vi "Read Index.vi"(3 "Index_Pointer)":refnum<class "Absolute_Pointer.lvclass">) -> (1 "Index Out":i32)   [LabVIEW 2020, in "Absolute_Pointer.lvclass"]
uses:
  Absolute_Pointer.lvclass
  Absolute_Pointer.lvclass/Absolute_Pointer.ctl
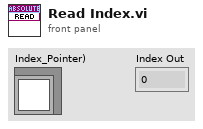
[diagram p1: front panel]
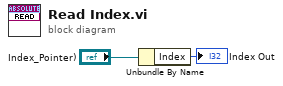
[diagram p0: block diagram]
diagram:
  n1 = Unbundle By Name("Index_Pointer)") -> ("Index"=→"Index Out":i32)
